vi "GetHistogram.vi"(0 "Image":T1, 7 "Mask":T1, 11 "error in":errorcluster) -> (4 "Waveform Graph":u32[](graph), 6 "Gray Level Intensities":T2 {"Standard  Deviation" format="%.2f"; "Mean Intensity" format="%.2f"; "Maximum Intensity" format="%.2f"; "Minimum Intensity" format="%.2f"}, 15 "error out":errorcluster)   [LabVIEW 2015]
uses:
  <vilib>/vision/Image Controls.llb/IMAQ Image.ctl
  <vilib>/vision/NI_Vision_Development_Module.lvlib
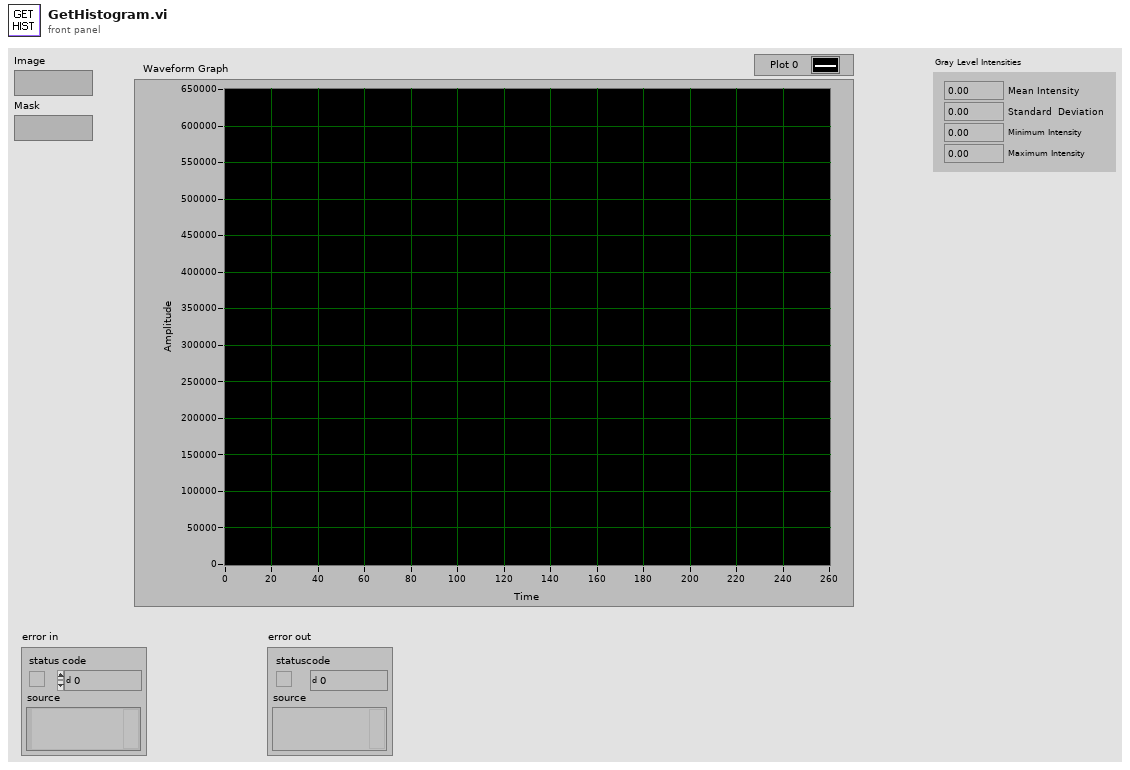
[diagram p1: front panel]
types:
  T1 = typedef "IMAQ Image.ctl" = refnum<image>
  T2 = cluster{"Mean Intensity":sgl, "Standard  Deviation":sgl, "Minimum Intensity":sgl, "Maximum Intensity":sgl}
  T3 = cluster{"histogram":u32[], "Minimal Value":sgl, "Maximal Value":sgl, "Starting Value":sgl, "Interval Width":sgl, "Mean Value":sgl, "Standard  Variation":sgl, "Area (pixels)":i32}
  T4 = cluster{"Mean Value":sgl, "Standard  Variation":sgl, "Minimal Value":sgl, "Maximal Value":sgl}
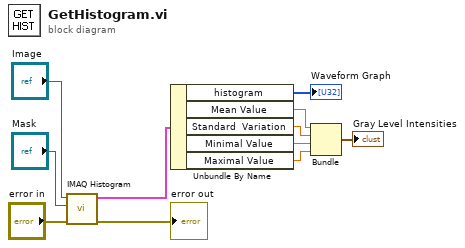
[diagram p0: block diagram]
diagram:
  n1 = call "IMAQ Histogram"("error in (no error)"="error in", "Image Mask"="Mask", "Image"="Image") -> ("error out"=→"error out":errorcluster, "Histogram Report"=w11:T3)  [unwired: 7 in]
  n2 = Unbundle By Name(w11) -> ("histogram"=→"Waveform Graph":u32[], "Mean Value"=w7:sgl, "Standard  Variation"=w6:sgl, "Minimal Value"=w5:sgl, "Maximal Value"=w4:sgl)
  n3 = Bundle("Mean Value"=w7, "Standard  Variation"=w6, "Minimal Value"=w5, "Maximal Value"=w4) -> (→"Gray Level Intensities":T4)  [unwired: 1 out]
